vi "initialize tree.vi"(8 "error in (no error)":errorcluster, 10 "TreeControl in":refnum<vi>, 11 "Node Ptr":T1 format="%.0x") -> (0 "error out":errorcluster, 3 "Item Ref out":T1 format="%.0x")   [LabVIEW 2016, in "FPGA Addon System Explorer.lvlib"]
uses:
  FPGA Addon System Explorer.lvlib
  <vilib>/NI Veristand/Custom Device API/Custom Device Item Ref.ctl
  reservation type.ctl
  <vilib>/NI VeriStand/Custom Device API/Custom Device API.lvlib
  FPGA RM Client API.lvlib
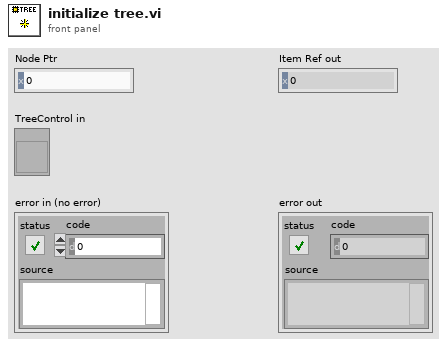
[diagram p1: front panel]
types:
  T1 = typedef "Custom Device API.lvlib/Custom Device Item Ref.ctl" = u64
  T2 = cluster{"Left Cell String":string, "Child Text":string[], "Child Tag":string, "Item Indent":i32, "Child Only?":bool, "Glyph Index":i32}[]
  T3 = typedef "FPGA Addon System Explorer.lvlib/reservation type.ctl" = enum16{"none", "available", "reserved by this", "reserved by other", "incompatible", "parent"}
  T4 = typedef "FPGA RM Client API.lvlib/fpga resource.ctl" = cluster{"name":string, "datatype":string, "channel type":T5, "value":variant, "notes":string}
  T5 = typedef "FPGA RM Client API.lvlib/Channel Type.ctl" = enum16{"Write Channel", "Read Channel", "Write Waveform", "Read Waveform"}
  T6 = cluster{"Left Cell String":string, "Child Text":string[], "Child Tag":string, "Item Indent":i32, "Child Only?":bool, "Glyph Index":i32}
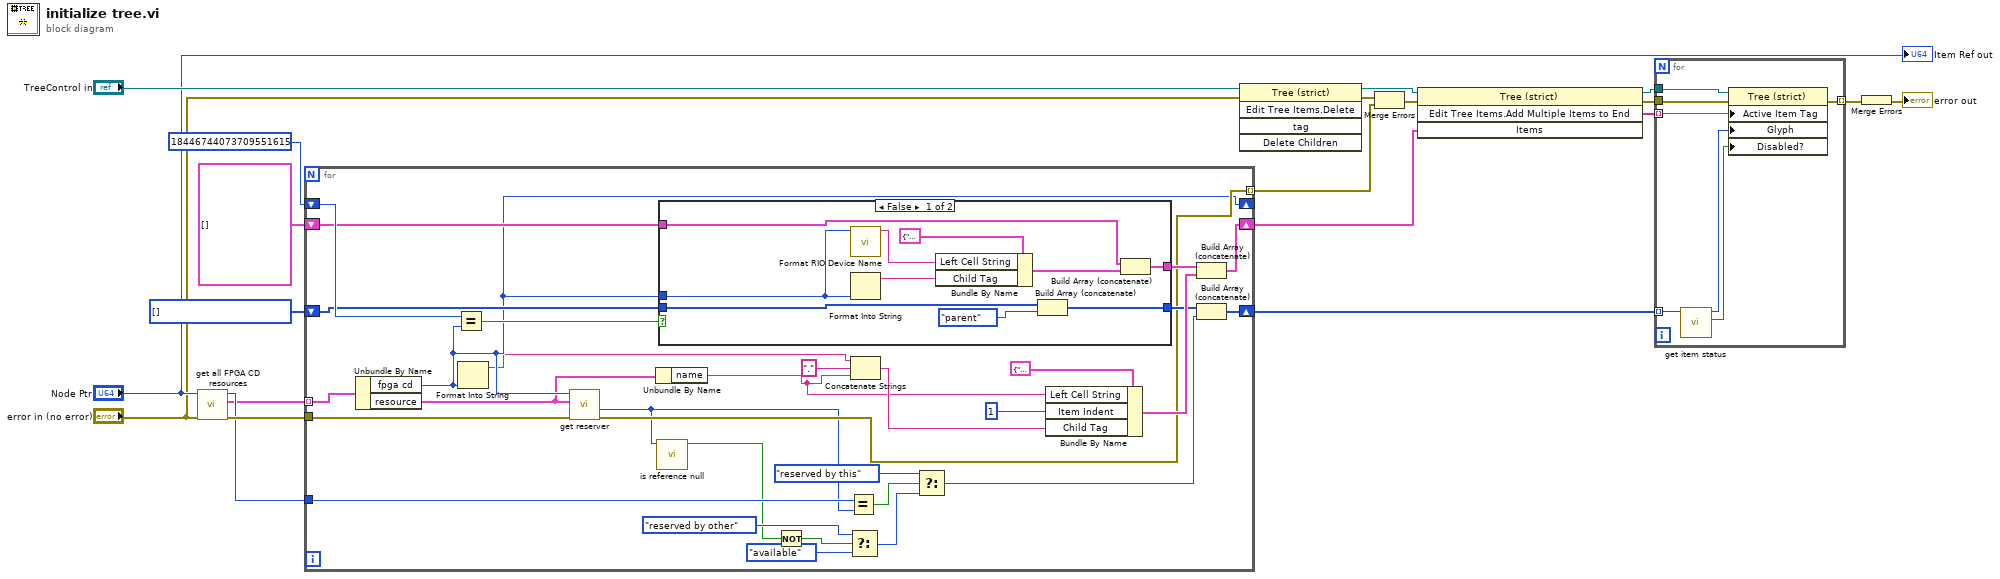
[diagram p0: block diagram]
diagram:
  w16 = T3[] [] items=["none", "available", "reserved by this", "reserved by other", "incompatible", "parent"]
  n1 = call "get all FPGA CD resources.vi"("error in (no error)"="error in (no error)", "Item Ref in"="Node Ptr") -> ("error out"=w9:errorcluster, "fpga resources"=w1:cluster{"fpga cd":T1, "resource":T4}[], "Item Ref out"=w2:T1)  [unwired: 7 in]
  n2 = for {
    tunnel: w1 -> [w50] mode=indexing
    shift-right: [w34] -> _
    shift-left: T1 18446744073709551615 ("FPGA CD Ref") -> [w48]
    shift-right: [w43] -> w14
    shift-left: T2 [] ("Item") -> [w46]
    shift-right: [w37] -> w12
    shift-left: w16 -> [w39]
    tunnel: w9 -> [w36]
    tunnel: [w35] -> w8 mode=indexing
    tunnel: w2 -> [w32]
    n3 = Unbundle By Name(w50) -> ("fpga cd"=w34:T1, "resource"=w25:T4)
    n4 = Equal?(x=w48, y=w34) -> (x = y?=w47:bool)
    n5 = Format Into String(w34) -> (resulting string=w33:string)  [unwired: 3 in, 1 out]
    n6 = call "get reserver.vi"("error in (no error)"=w36, "FPGA Resource"=w25, "Item Ref in"=w34) -> ("error out"=w35:errorcluster, "Dependent Node Ref"=w24:T1)  [unwired: 6 in, 1 out]
    n7 = Unbundle By Name(w25) -> ("name"=w21:string)
    n8 = call "is reference null.vi"("reserver"=w24) -> ("Boolean"=w23:bool)  [unwired: 10 in]
    n9 = case shown="False" w47 {
      tunnel: w34 -> [w59 _]
      tunnel: w46 -> [w57 w62]
      tunnel: [w55 w62] -> w45
      tunnel: w39 -> [w53 w61]
      tunnel: [w52 w61] -> w38
      frame False {
        n10 = call "Format RIO Device Name.vi"("FPGA CD Ref"=w59) -> ("String"=w54:string)  [unwired: 9 in, 1 out]
        n11 = Format Into String(w59) -> (resulting string=w58:string)  [unwired: 3 in, 1 out]
        n12 = Bundle By Name(cluster=T6 {"Left Cell String"="", "Child Text"=[], "Child Tag"="", "Item Indent"=0, "Child Only?"=FALSE, "Glyph Index"=0} ("Item"), "Left Cell String"=w54, "Child Tag"=w58) -> (w56:T6)
        n13 = Build Array (concatenate)(w53, reservation_type."parent" ("element")) -> (w52:T3[])
        n14 = Build Array (concatenate)(w57, w56) -> (w55:T2)
      }
      frame True {
      }
    }
    n15 = Not(x=w23) -> (.not. x?=w22:bool)
    n16 = Equal?(x=w32, y=w24) -> (x = y?=w31:bool)
    n17 = Select(t=reservation_type."reserved by other" ("element"), s=w22, f=reservation_type."available" ("element")) -> (s? t:f=w27:T3)
    n18 = Concatenate Strings(w33, "." ("string"), w21) -> (w40:string)
    n19 = Select(t=reservation_type."reserved by this" ("element"), s=w31, f=w27) -> (s? t:f=w26:T3)
    n20 = Bundle By Name(cluster=T6 {"Left Cell String"="", "Child Text"=[], "Child Tag"="", "Item Indent"=0, "Child Only?"=FALSE, "Glyph Index"=0} ("Item"), "Left Cell String"=w21, "Item Indent"=1, "Child Tag"=w40) -> (w44:T6)
    n21 = Build Array (concatenate)(w45, w44) -> (w43:T2)
    n22 = Build Array (concatenate)(w38, w26) -> (w37:T3[])
  }
  n23 = invoke on="Invoke Node" class="Tree (strict)" method="Edit Tree Items.Delete"(reference="TreeControl in", error in="error in (no error)") -> (reference out=w15:refnum<vi>, error out=w7:errorcluster)  [unwired: 3 in, 3 out]
  n24 = Merge Errors(w7, w8) -> (w6:errorcluster)
  n25 = invoke on="Invoke Node" class="Tree (strict)" method="Edit Tree Items.Add Multiple Items to End"(reference=w15, error in=w6, "Items"=w14) -> (reference out=w11:refnum<vi>, error out=w5:errorcluster, "Edit Tree Items:Add Multiple Items to End"=w13:string[])  [unwired: 1 in, 1 out]
  n26 = for {
    tunnel: w13 -> [w69] mode=indexing
    tunnel: w12 -> [w68] mode=indexing
    tunnel: w11 -> [w65]
    tunnel: w5 -> [w64]
    tunnel: [w63] -> w4 mode=indexing
    n27 = call "get item status.vi"("element"=w68) -> ("Disabled?"=w66:bool, "symbol index"=w67:i32)  [unwired: 9 in]
    n28 = property class="Tree (strict)"(reference=w65, error in=w64, "Active Item Tag"=w69, "Glyph"=w67, "Disabled?"=w66) -> (error out=w63:errorcluster)  [unwired: 1 out]
  }
  n29 = Merge Errors(w4) -> (→"error out":errorcluster)
  "Item Ref out" <- "Node Ptr"
